vi "FPGA_AnalogTriggerOpen.vi"(8 "error in":errorcluster, 11 "AnalogTriggerChannel":T2=enum."Invalid") -> (0 "error out":errorcluster, 3 "AnalogTriggerDevRef":T1)   [LabVIEW 2017]
uses:
  <vilib>/Rock Robotics/SystemInterfaces/AnalogTrigger/FPGA_AnalogTriggerIndex.ctl
  <vilib>/Rock Robotics/SystemInterfaces/AnalogTrigger/FPGA_AnalogTriggerDevRef.ctl
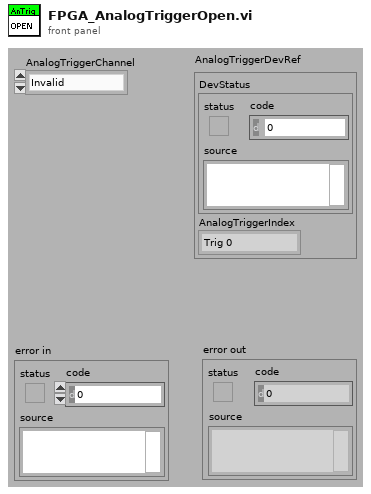
[diagram p1: front panel]
types:
  T1 = typedef "FPGA_AnalogTriggerDevRef.ctl" = cluster{"DevStatus":errorcluster, "AnalogTriggerIndex":T2}
  T2 = typedef "FPGA_AnalogTriggerIndex.ctl" = enum8{"Trig 0", "Trig 1", "Trig 2", "Trig 3", "Trig 4", "Trig 5", "Trig 6", "Trig 7", "Invalid"}
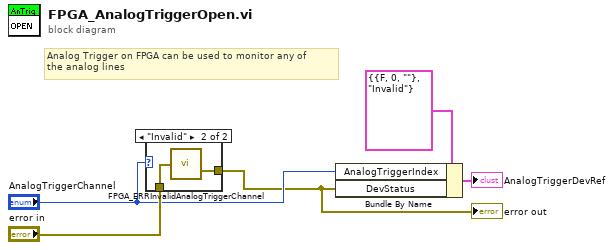
[diagram p0: block diagram]
diagram:
  # "Analog Trigger on FPGA can be used to monitor any of\nthe analog lines"
  n1 = case shown="\"Invalid\"" "AnalogTriggerChannel" {
    tunnel: [w6 w8] -> w1
    tunnel: "error in" -> [w6 w7]
    frame Default {
    }
    frame "Invalid" {
      n2 = call <vilib>:"FPGA_ERRInvalidAnalogTriggerChannel.vi"("error in (no error)"=w7) -> ("error out"=w8:errorcluster)
    }
  }
  "error out" <- w1
  n3 = Bundle By Name(cluster=T1 {"DevStatus"={"status"=FALSE, "code"=0, "source"=""}, "AnalogTriggerIndex"=enum."Invalid"} ("AnalogTriggerDevRef"), "AnalogTriggerIndex"="AnalogTriggerChannel", "DevStatus"=w1) -> (→"AnalogTriggerDevRef":T1)
